vi "SDI_Dual-Axis_Test.vi"() -> ()   [LabVIEW 2014]
uses:
  <vilib>/Motion/plugins/PluginFramework/nismSDIFramework.SetFrameworkMode.multi.vi
  <vilib>/Motion/Express/_s/nimc.ex.clearFaults.clearFaults.axis.vi
  <vilib>/Motion/Express/_s/nimc.ex.power.power.axis.vi
  <vilib>/Motion/BlockNode/FB.NIMotion.xnode
  <vilib>/Motion/plugins/Delta ASDA SDI Plug-in/Template SoftMotion Drive Interface Plug-in Class.lvclass
panel:
  in  "stop":bool
  out "error out":errorcluster
  in  "Axis 2":refnum<k21>="Axis 2"
  in  "Axis":refnum<k21>="Axis 1"
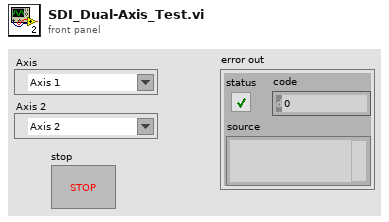
[diagram p1: front panel]
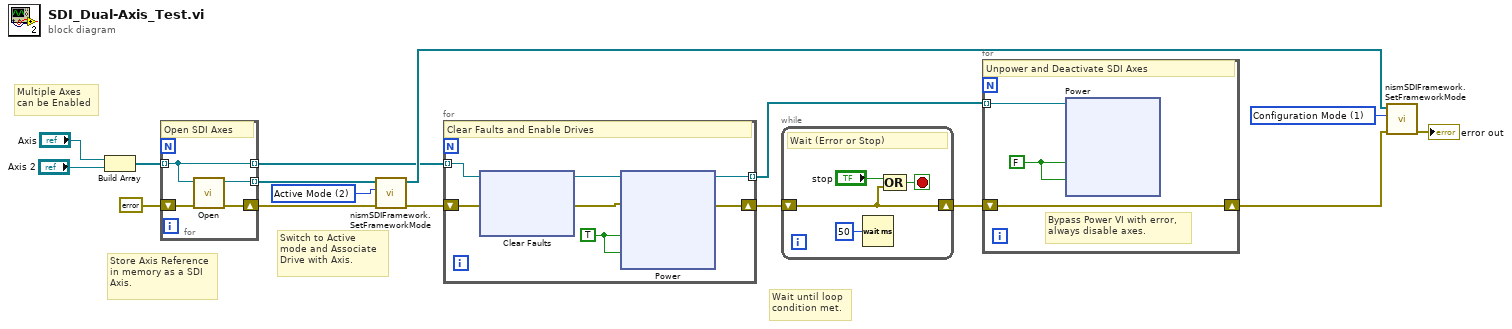
[diagram p0: block diagram]
diagram:
  w12 = 2 items=["Configuration Mode"=1, "Active Mode"=2] ("mode (Active Mode)")
  w16 = 1 items=["Configuration Mode"=1, "Active Mode"=2] ("mode (Active Mode)")
  # "Wait until loop\ncondition met."
  # "Store Axis Reference\nin memory as a SDI\nAxis."
  # "Switch to Active\nmode and Associate\nDrive with Axis."
  # "Multiple Axes\ncan be Enabled"
  n1 = Build Array("Axis", "Axis 2") -> (w10:refnum<k21>[])
  n2 = for {
    tunnel: w10 -> [w17] mode=indexing
    tunnel: [w20] -> w9 mode=indexing
    shift-right: [w19] -> w8
    shift-left: errorcluster {"status"=FALSE, "code"=0, "source"=""} ("error out") -> [w18]
    tunnel: [w17] -> w1 mode=indexing
    # "Open SDI Axes"
    n3 = call <vilib>:"Open.vi"("error in (no error)"=w18, "Axis"=w17) -> ("error out"=w19:errorcluster, "Base Axis Out"=w20:refnum<class "nismPluginAxisBaseClass.lvclass">)  [unwired: 8 in]
  }
  n4 = call-poly <vilib>:"nismSDIFramework.SetFrameworkMode.vi"("error in (no error)"=w8, "mode (Active Mode)"=w12, "Base Axis In"=w9) -> ("error out"=w11:errorcluster, "Base Axis Out"=w6:refnum<class "nismPluginAxisBaseClass.lvclass">[])  [unwired: 7 in]
  n5 = for {
    tunnel: w1 -> [w23] mode=indexing
    tunnel: [w22] -> w2 mode=indexing
    shift-right: [w25] -> w3
    shift-left: w11 -> [w24]
    w27 = TRUE ("enable axis")
    # "Clear Faults and Enable Drives"
    n6 = xnode ("Clear Faults")("resource"=w23, "error in"=w24) -> ("resource out"=w21:refnum<k21>, "error out"=w26:errorcluster)
    n7 = xnode ("Power")("enable axis"=w27, "enable drive"=w27, "resource"=w21, "error in"=w26) -> ("resource out"=w22:refnum<k21>, "error out"=w25:errorcluster)
  }
  n8 = while {
    shift-right: [w42] -> w13
    shift-left: w3 -> [w42]
    stop <- w44 stop-if-true
    # "Wait (Error or Stop)"
    n9 = Wait (ms)(milliseconds to wait=u32 50) -> ()  [unwired: 1 out]
    n10 = Compound Arithmetic op=OR("stop", w42) -> (w44:bool)
  }
  n11 = for {
    tunnel: w2 -> [w47] mode=indexing
    shift-right: [w46] -> w15
    shift-left: w13 -> [w46]
    w48 = FALSE ("enable axis")
    # "Bypass Power VI with error,\nalways disable axes."
    # "Unpower and Deactivate SDI Axes"
    n12 = xnode ("Power")("enable axis"=w48, "enable drive"=w48, "resource"=w47) -> ()  [unwired: 1 in, 2 out]
  }
  n13 = call-poly <vilib>:"nismSDIFramework.SetFrameworkMode.vi"("error in (no error)"=w15, "mode (Active Mode)"=w16, "Base Axis In"=w6) -> ("error out"=→"error out":errorcluster)  [unwired: 7 in, 1 out]
